vi "Compensa Roda Rápido.vi"() -> ()   [LabVIEW 2016]
uses:
  <vilib>/Analysis/Matrix/Datatypes/RealMatrix.ctl
  <vilib>/Analysis/Matrix/Numeric/Conversions/Array To Matrix - RA.vi
  <vilib>/Analysis/Matrix/Numeric/Absolute Value/Absolute Value - RM.vi
  <vilib>/Analysis/Matrix/Numeric/Multiply/Multiply - RM,RM.vi
  <vilib>/Analysis/Matrix/NI_Matrix.lvlib
panel:
  out "Motor a sobrescrever velocidade":bool[][](array[boolean])
  out "Velocidade Necessária Motores":T1
  in  "Velocidade das Rodas Lido":dbl[](array[numeric])=[0.866025, -0.866025, -0.707107, 0.1]
  in  "Velocidade do Robô Desejada":dbl[](array[numeric])=[0.0, 1.0, 0.0]
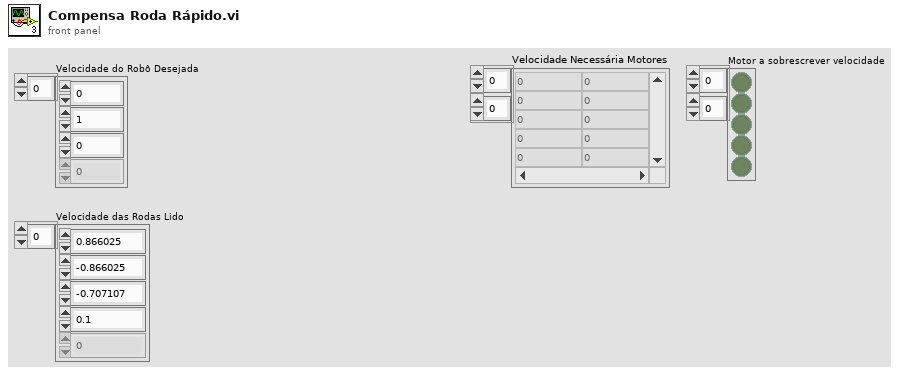
[diagram p1: front panel]
types:
  T1 = typedef "NI_Matrix.lvlib/RealMatrix.ctl" = dbl[][]
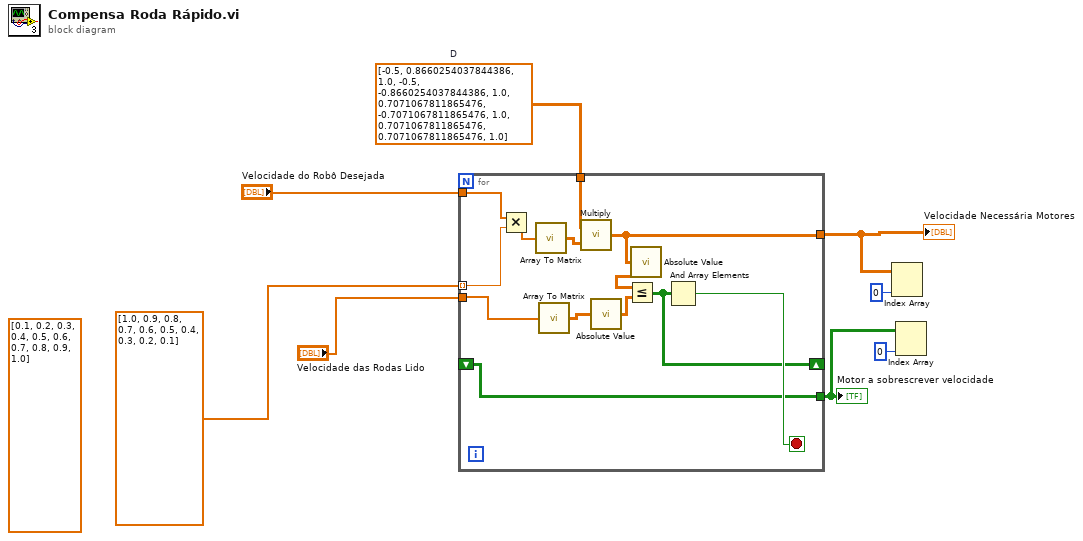
[diagram p0: block diagram]
diagram:
  w6 = T1 [[-0.5, 0.8660254037844386, 1.0], [-0.5, -0.8660254037844386, 1.0], [0.7071067811865476, -0.7071067811865476, 1.0], [0.7071067811865476, 0.7071067811865476, 1.0]]  # D
  (unwired) dbl[] [0.1, 0.2, 0.3, 0.4, 0.5, 0.6, 0.7, 0.8, 0.9, 1.0] ("reversed array")
  n1 = for {
    tunnel: "Velocidade do Robô Desejada" -> [w21]
    tunnel: dbl[] [1.0, 0.9, 0.8, 0.7, 0.6, 0.5, 0.4, 0.3, 0.2, 0.1] -> [w20] mode=indexing
    tunnel: w6 -> [w19]
    tunnel: "Velocidade das Rodas Lido" -> [w16]
    tunnel: [w14] -> w3
    shift-right: [w10] -> _
    shift-left: _ -> [w9]
    tunnel: [w9] -> w5
    stop <- w15 stop-if-true
    n2 = Multiply(x=w21, y=w20) -> (x*y=w18:dbl[])
    n3 = call-poly <vilib>:"Array To Matrix.vi"("Real 1D Array"=w18) -> ("Real Matrix (Column Vector)"=w17:T1)
    n4 = call-poly <vilib>:"Array To Matrix.vi"("Real 1D Array"=w16) -> ("Real Matrix (Column Vector)"=w12:T1)
    n5 = call-poly <vilib>:"Multiply.vi"("Real Matrix B"=w17, "Real Matrix A"=w19) -> ("A * B"=w14:T1)
    n6 = call-poly <vilib>:"Absolute Value.vi"("Real Matrix A"=w12) -> ("|A|"=w11:T1)
    n7 = call-poly <vilib>:"Absolute Value.vi"("Real Matrix A"=w14) -> ("|A|"=w13:T1)
    n8 = Less Or Equal?(x=w13, y=w11) -> (x <= y?=w10:bool[][])
    n9 = And Array Elements(Boolean array=w10) -> (logical AND=w15:bool)
  }
  "Velocidade Necessária Motores" <- w3
  "Motor a sobrescrever velocidade" <- w5
  n10 = Index Array(array=w3, index (col)=0 ("disabled index (col)")) -> ()  [unwired: 1 in, 1 out]
  n11 = Index Array(array=w5, index (col)=0 ("disabled index (col)")) -> ()  [unwired: 1 in, 1 out]
